vi "例6-5.vi"() -> ()   [LabVIEW 2019]
uses:
  <vilib>/measure/NI_MAPro.lvlib
panel:
  out "波形图":waveform(dbl)(graph)
  in  "采样点数":dbl=1000.0
  in  "采样频率":dbl=1000.0
  in  "公式":string="sin(w*t)/(w*t)"
  in  "幅值":dbl=1.0
  in  "频率":dbl=5.0
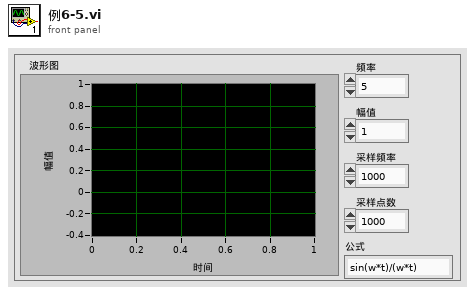
[diagram p1: front panel]
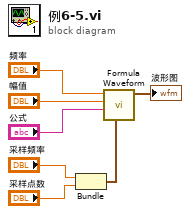
[diagram p0: block diagram]
diagram:
  n1 = Bundle("采样频率"="采样频率", "采样点数"="采样点数") -> (w2:cluster{"采样频率":dbl, "采样点数":dbl})  [unwired: 1 in]
  n2 = call <vilib>:"Formula Waveform.vi"("sampling info"=w2, "formula"="公式", "amplitude"="幅值", "frequency"="频率") -> ("signal out"=→"波形图":waveform(dbl))  [unwired: 6 in, 1 out]
